vi "Weather Station UI.vi"(10 "하위 리미트":dbl=10.0, 11 "상위 리미트":dbl=30.0) -> (1 "경고":string, 2 "온도 히스토리":dbl(graph))   [LabVIEW 2010]
doc: "이것은 기상 관측기 프로젝트의 메인 VI입니다. 온도와 바람 경고 시스템을 위한 사용자 인터페이스를 가지고 있습니다. \n\n사용자 입력: 상위 리미트, 하위 리미트, 최대 풍속.\n출력: 온도 히스토리 차트, 풍속 히스토리 차트, 경고 문자열."
uses:
  Supporting Files/Weather Station States.ctl
panel:
  in  "날씨 데이터":dynamicdata(graph)
  in  "정지":bool
  in  "풍속 상위 리미트":dbl(slide)=50.0 scale=0.0..100.0
  out "풍속 히스토리":dbl(graph)
  # "섭씨"
  # "온도 범위 (C)"
  # "열사병"
  # "동상"
  # "kph"
  # "최대 안전 풍속 (kph)"
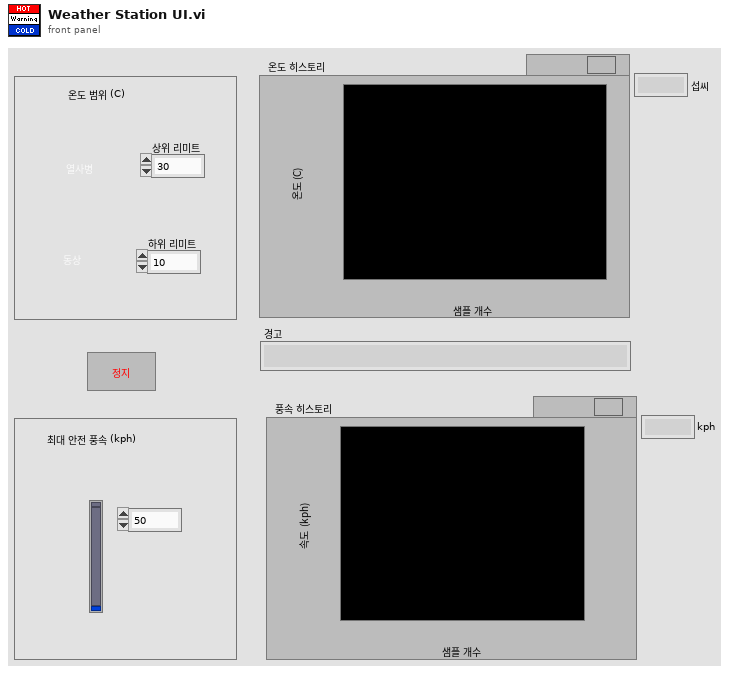
[diagram p1: front panel]
types:
  T1 = cluster{"Temperature":dbl, "T Upper Limit":dbl, "T Lower Limit":dbl, "Wind Speed":dbl, "Wind Upper Limit":dbl, "Warning":string, "Time":dbl}
  T2 = typedef "Weather Station States.ctl" = enum16{"분석", "UI 처리", "경고 설정", "데이터 로그", "정지"}
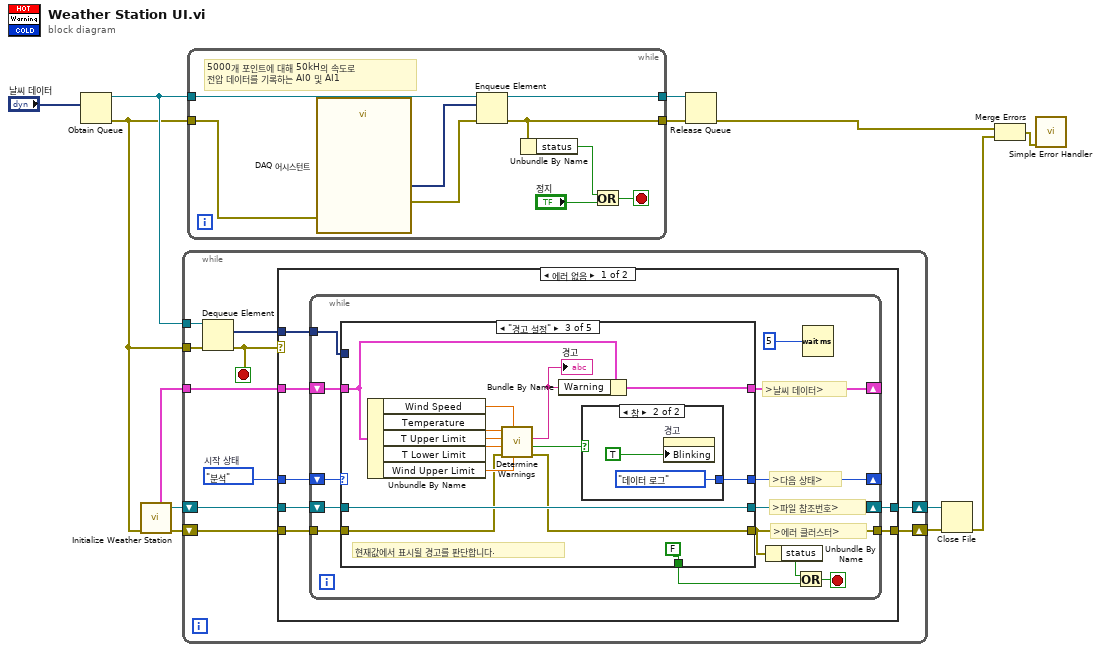
[diagram p0: block diagram]
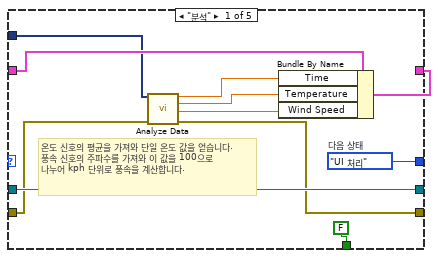
[diagram p2: hidden frame]
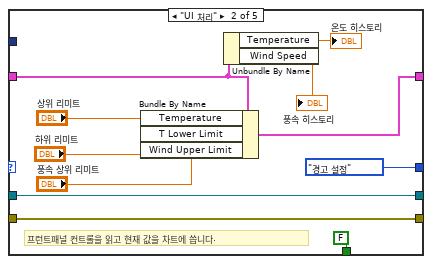
[diagram p3: hidden frame]
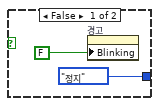
[diagram p4: hidden frame]
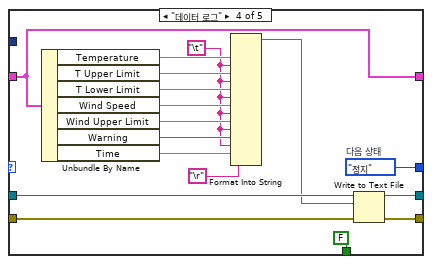
[diagram p5: hidden frame]
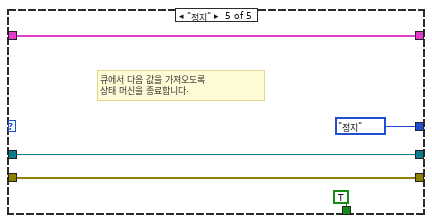
[diagram p6: hidden frame]
diagram:
  n1 = Obtain Queue(element data type="날씨 데이터") -> (queue out=w10:refnum<queue>, error out=w1:errorcluster)  [unwired: 4 in, 1 out]
  n2 = call "Initialize Weather Station.vi"("에러 입력(에러 없음)"=w1) -> ("에러 출력"=w2:errorcluster, "파일 참조번호"=w3:refnum<file>, "날씨 데이터"=w13:T1)  [unwired: 8 in]
  n3 = while {
    tunnel: w13 -> [w22]
    tunnel: w10 -> [w21]
    tunnel: w1 -> [w20]
    shift-right: [w23] -> w6
    shift-left: w3 -> [w19]
    shift-right: [w15] -> w5
    shift-left: w2 -> [w16]
    stop <- w18 stop-if-true
    w14 = Weather_Station_States."분석"  # 시작 상태
    n4 = Dequeue Element(queue=w21, error in (no error)=w20) -> (element=w17:dynamicdata, error out=w18:errorcluster)  [unwired: 1 in, 2 out]
    n5 = case shown="에러 없음" w18 {
      tunnel: [w30 w106] -> w23
      tunnel: w22 -> [w29 _]
      tunnel: w19 -> [w28 w106]
      tunnel: w17 -> [w27 _]
      tunnel: w16 -> [w25 w107]
      tunnel: [w26 w107] -> w15
      tunnel: w14 -> [w24 _]
      frame No Error {
        n6 = while {
          shift-right: [w43] -> _
          shift-left: w24 -> [w35]
          shift-right: [w32] -> w30
          shift-left: w28 -> [w42]
          shift-right: [w36] -> _
          shift-left: w29 -> [w39]
          tunnel: w27 -> [w34]
          tunnel: [w33] -> w26
          tunnel: w25 -> [w31]
          stop <- w41 stop-if-true
          # ">에러 클러스터>"
          # ">날씨 데이터>"
          # ">파일 참조번호>"
          # ">다음 상태>"
          n7 = case shown="\"경고 설정\"" w35 {
            tunnel: [w54 Weather_Station_States."경고 설정" ("Next State") w78 w100 Weather_Station_States."정지" ("Next State")] -> w43
            tunnel: [w44 w57 w68 w97 w101] -> w33
            tunnel: w42 -> [w50 w56 w75 w96 w102]
            tunnel: [w51 w65 w76 w94 w103] -> w36
            tunnel: w39 -> [w52 w63 w77 w94 w103]
            tunnel: [FALSE ("stop") FALSE ("stop") FALSE ("stop") FALSE ("stop") TRUE ("stop")] -> w38
            tunnel: w34 -> [w49 _ _ _ _]
            tunnel: [w50 w56 w75 w98 w102] -> w32
            tunnel: w31 -> [w48 w57 w69 w84 w101]
            frame "분석" {
              w54 = Weather_Station_States."UI 처리"  # 다음 상태
              # "온도 신호의 평균을 가져와 단일 온도 값을 얻습니다. 풍속 신호의 주파수를 가져와 이 값을 100으로 나누어 kph 단위로 풍속을 계산합니다."
              n8 = call "Analyze Data.vi"("날씨 데이터"=w49, "에러 입력"=w48) -> ("시간"=w47:dbl, "온도"=w46:dbl, "풍속"=w45:dbl, "에러 출력"=w44:cluster{"상태":bool, "코드":i32, "소스":string})  [unwired: 10 in]
              n9 = Bundle By Name(cluster=w52, "Time"=w47, "Temperature"=w46, "Wind Speed"=w45) -> (w51:T1)
            }
            frame "UI 처리" {
              # "프런트패널 컨트롤을 읽고 현재 값을 차트에 씁니다."
              n10 = Bundle By Name(cluster=w63, "Temperature"="상위 리미트", "T Lower Limit"="하위 리미트", "Wind Upper Limit"="풍속 상위 리미트") -> (w65:T1)
              n11 = Unbundle By Name(w63) -> ("Temperature"=→"온도 히스토리":dbl, "Wind Speed"=→"풍속 히스토리":dbl)
            }
            frame "경고 설정" {
              # "현재값에서 표시될 경고를 판단합니다."
              n12 = Unbundle By Name(w77) -> ("Wind Speed"=w74:dbl, "Temperature"=w73:dbl, "T Upper Limit"=w72:dbl, "T Lower Limit"=w71:dbl, "Wind Upper Limit"=w70:dbl)
              n13 = call "Determine Warnings.vi"("최대 풍속"=w70, "현재 풍속"=w74, "에러 입력 (에러 없음)"=w69, "최저 온도"=w71, "최고 온도"=w72, "현재 온도"=w73) -> ("에러 출력"=w68:cluster{"상태":bool, "코드":i32, "소스":string}, "경고?"=w67:bool, "경고 텍스트"=w66:string)  [unwired: 3 in]
              "경고" <- w66
              n14 = Bundle By Name(cluster=w77, "Warning"=w66) -> (w76:T1)
              n15 = case shown="참" w67 {
                tunnel: [Weather_Station_States."정지" ("Next State") Weather_Station_States."데이터 로그" ("Next State")] -> w78
                frame False {
                  n16 = property on="경고" class="Str"("Blinking"=FALSE) -> ()  [unwired: 2 in, 2 out]
                }
                frame True {
                  n17 = property on="경고" class="Str"("Blinking"=TRUE) -> ()  [unwired: 2 in, 2 out]
                }
              }
            }
            frame "데이터 로그" {
              w86 = "\t"
              w100 = Weather_Station_States."정지"  # 다음 상태
              n18 = Unbundle By Name(w94) -> ("Temperature"=w93:dbl, "T Upper Limit"=w92:dbl, "T Lower Limit"=w91:dbl, "Wind Speed"=w90:dbl, "Wind Upper Limit"=w89:dbl, "Warning"=w88:string, "Time"=w87:dbl)
              n19 = Format Into String(w93, w86, w92, w86, w91, w86, w90, w86, w89, w86, w88, w86, w87, "\r") -> (resulting string=w95:string)  [unwired: 3 in, 1 out]
              n20 = Write to Text File(file (use dialog)=w96, text=w95, error in=w84) -> (refnum out=w98:refnum<file>, error out=w97:errorcluster)  [unwired: 1 in, 1 out]
            }
            frame "정지" {
              # "큐에서 다음 값을 가져오도록\n상태 머신을 종료합니다."
            }
          }
          n21 = Unbundle By Name(w33) -> ("status"=w40:bool)
          n22 = Or(x=w40, y=w38) -> (x .or. y?=w41:bool)
          n23 = Wait (ms)(milliseconds to wait=u32 5 ("y")) -> ()  [unwired: 1 out]
        }
      }
      frame Error {
      }
    }
  }
  n24 = while {
    tunnel: w10 -> [w116]
    tunnel: w1 -> [w110]
    tunnel: [w113] -> w12
    tunnel: [w115] -> w11
    stop <- w111 stop-if-true
    # "5000개 포인트에 대해 50kH의 속도로 \n전압 데이터를 기록하는 AI0 및 AI1"
    n25 = call "DAQ 어시스턴트"("error in"=w110) -> ("data"=w108:dynamicdata, "error out"=w109:errorcluster)  [unwired: 16 in, 1 out]
    n26 = Enqueue Element(queue=w116, element=w108, error in (no error)=w109) -> (queue out=w115:refnum<queue>, error out=w113:errorcluster)  [unwired: 1 in, 1 out]
    n27 = Unbundle By Name(w113) -> ("status"=w112:bool)
    n28 = Or(x=w112, y="정지") -> (x .or. y?=w111:bool)
  }
  n29 = Release Queue(queue=w11, error in (no error)=w12) -> (error out=w8:errorcluster)  [unwired: 1 in, 2 out]
  n30 = Close File(refnum=w6, error in=w5) -> (error out=w4:errorcluster)  [unwired: 1 out]
  n31 = Merge Errors(w8, w4) -> (w7:errorcluster)
  n32 = call <vilib>:"Simple Error Handler.vi"("error in (no error)"=w7) -> ()  [unwired: 4 in, 5 out]
